vi "camera_acq_H_noshutter_sub.vi"(5 "Shutter time (ms)":dbl, 7 "Exposure time (ms)":dbl, 8 "error in (no error)":errorcluster, 9 "Binning":dbl=1.0 format="%#_13g", 10 "Camera in":u32, 11 "VISA in":refnum<visa-resource-name>) -> (0 "error out":errorcluster, 1 "Image":u16[][](graph), 2 "Camera out":u32, 3 "VISA out":refnum<visa-resource-name>)   [LabVIEW 2018]
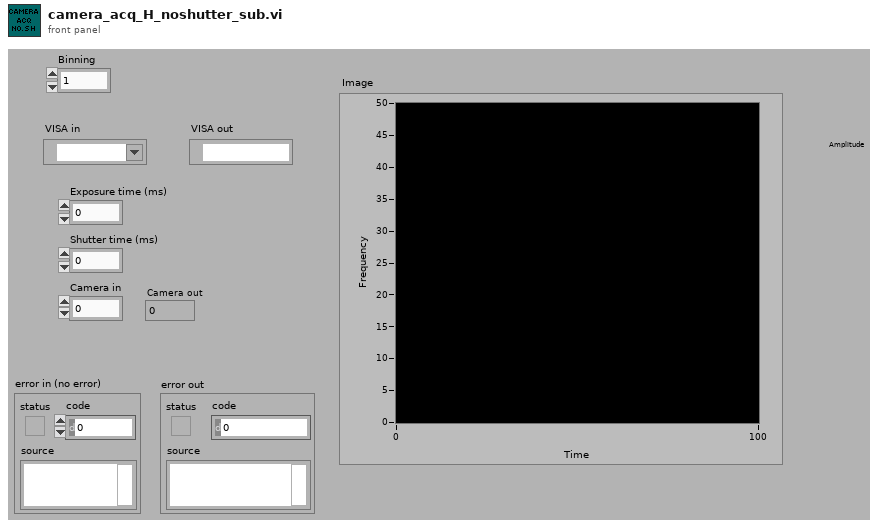
[diagram p1: front panel]
types:
  T1 = enum16{"Fast-mode", "Soft-mode", "Neutral Density"}
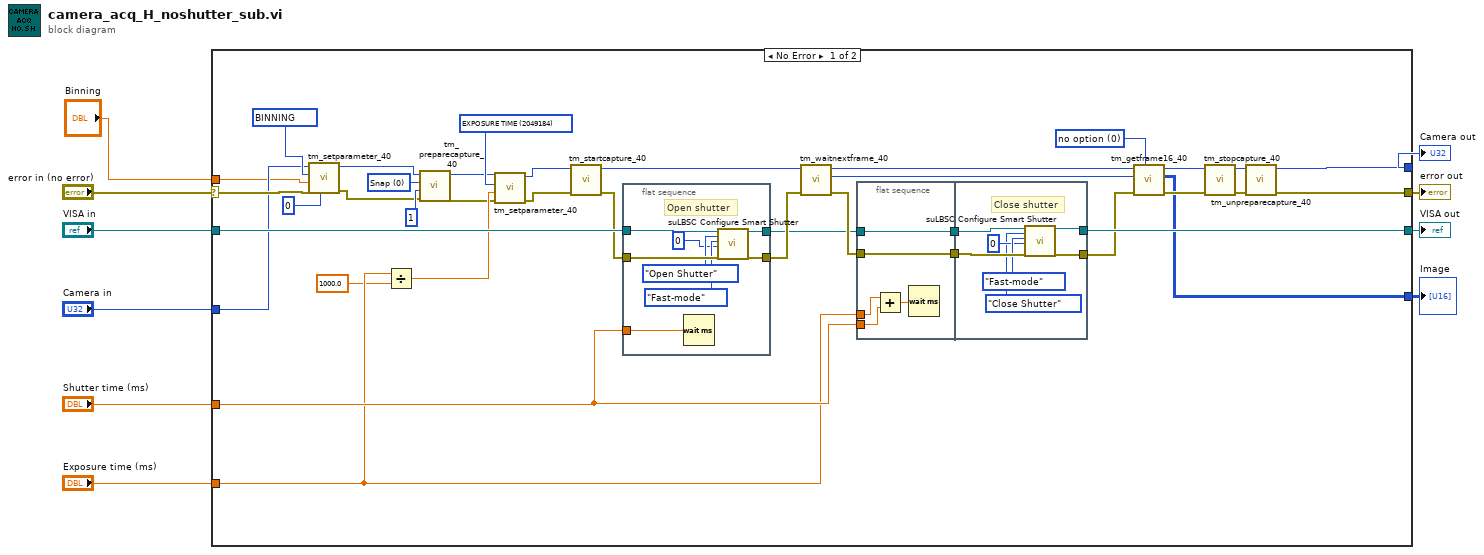
[diagram p0: block diagram]
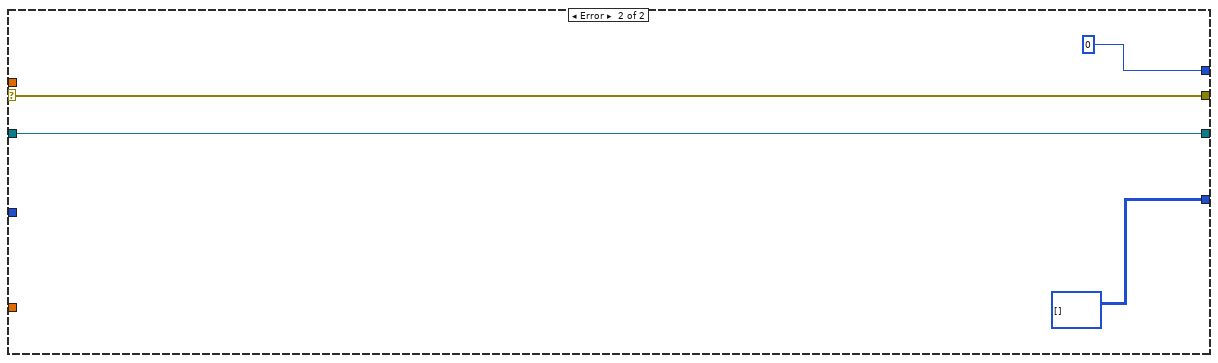
[diagram p2: hidden frame]
diagram:
  n1 = case shown="No Error" "error in (no error)" {
    selector: "error in (no error)" -> [w19 w71]
    tunnel: "Exposure time (ms)" -> [w31 _]
    tunnel: [w22 u32 0 ("Handle out")] -> w8
    tunnel: "VISA in" -> [w45 w72]
    tunnel: "Shutter time (ms)" -> [w44 _]
    tunnel: [w36 w71] -> w10
    tunnel: [w43 w72] -> w4
    tunnel: "Camera in" -> [w18 _]
    tunnel: [w32 u16[][] [] ("Data")] -> w2
    tunnel: "Binning" -> [w11 _]
    frame No Error {
      w16 = 0 items=["Snap", "Sequence"] ("Capture mode")
      w21 = u32 4215968 items=["SENSOR MODE"=4212128, "READOUT SPEED"=4211872, "READOUT DIRECTION"=4211904, "TRIGGER GLOBAL EXPOSURE"=2049680, "TRIGGER DELAY"=1066480, "INTERNAL TRIGGER HANDLING"=1066496, "SYNC READOUT SYSTEM BLANK"=1066528, "SENSOR TEMPERATURE"=2115232, "SENSOR COOLER STATUS"=2115280, "EXPOSURE TIME"=2049184, "DEFECT CORRECT MODE"=4670368, "BINNING"=4215968, "INTERNAL LINE SPEED"=4226000, "INTERNAL LINE INTERVAL"=4226016, "NUMBER OF OUTPUT TRIGGER CONNECTOR"=1852320, "OUTPUT TRIGGER SOURCE[0]"=1852576, "OUTPUT TRIGGER SOURCE[1]"=1852832, "OUTPUT TRIGGER SOURCE[2]"=1853088, "OUTPUT TRIGGER POLARITY[0]"=1852592, "OUTPUT TRIGGER POLARITY[1]"=1852848, "OUTPUT TRIGGER POLARITY[2]"=1853104, "OUTPUT TRIGGER ACTIVE[0]"=1852608, "OUTPUT TRIGGER ACTIVE[1]"=1852864, "OUTPUT TRIGGER ACTIVE[2]"=1853120, "OUTPUT TRIGGER DELAY[0]"=1852624, "OUTPUT TRIGGER DELAY[1]"=1852880, "OUTPUT TRIGGER DELAY[2]"=1853136, "OUTPUT TRIGGER PERIOD[0]"=1852640, "OUTPUT TRIGGER PERIOD[1]"=1852896, "OUTPUT TRIGGER PERIOD[2]"=1853152, "OUTPUT TRIGGER KIND[0]"=1852656, "OUTPUT TRIGGER KIND[1]"=1852912, "OUTPUT TRIGGER KIND[2]"=1853168, "OUTPUT TRIGGER BASE SENSOR[0]"=1852672, "OUTPUT TRIGGER BASE SENSOR[1]"=1852928, "OUTPUT TRIGGER BASE SENSOR[2]"=1853184, "OUTPUT TRIGGER PRE HSYNC COUNT"=1852704] ("Parameter")
      w26 = 0 items=["no option"=0, "high contrast"=16] ("Options")
      w42 = u32 2049184 items=["SENSOR MODE"=4212128, "READOUT SPEED"=4211872, "READOUT DIRECTION"=4211904, "TRIGGER GLOBAL EXPOSURE"=2049680, "TRIGGER DELAY"=1066480, "INTERNAL TRIGGER HANDLING"=1066496, "SYNC READOUT SYSTEM BLANK"=1066528, "SENSOR TEMPERATURE"=2115232, "SENSOR COOLER STATUS"=2115280, "EXPOSURE TIME"=2049184, "DEFECT CORRECT MODE"=4670368, "BINNING"=4215968, "INTERNAL LINE SPEED"=4226000, "INTERNAL LINE INTERVAL"=4226016, "NUMBER OF OUTPUT TRIGGER CONNECTOR"=1852320, "OUTPUT TRIGGER SOURCE[0]"=1852576, "OUTPUT TRIGGER SOURCE[1]"=1852832, "OUTPUT TRIGGER SOURCE[2]"=1853088, "OUTPUT TRIGGER POLARITY[0]"=1852592, "OUTPUT TRIGGER POLARITY[1]"=1852848, "OUTPUT TRIGGER POLARITY[2]"=1853104, "OUTPUT TRIGGER ACTIVE[0]"=1852608, "OUTPUT TRIGGER ACTIVE[1]"=1852864, "OUTPUT TRIGGER ACTIVE[2]"=1853120, "OUTPUT TRIGGER DELAY[0]"=1852624, "OUTPUT TRIGGER DELAY[1]"=1852880, "OUTPUT TRIGGER DELAY[2]"=1853136, "OUTPUT TRIGGER PERIOD[0]"=1852640, "OUTPUT TRIGGER PERIOD[1]"=1852896, "OUTPUT TRIGGER PERIOD[2]"=1853152, "OUTPUT TRIGGER KIND[0]"=1852656, "OUTPUT TRIGGER KIND[1]"=1852912, "OUTPUT TRIGGER KIND[2]"=1853168, "OUTPUT TRIGGER BASE SENSOR[0]"=1852672, "OUTPUT TRIGGER BASE SENSOR[1]"=1852928, "OUTPUT TRIGGER BASE SENSOR[2]"=1853184, "OUTPUT TRIGGER PRE HSYNC COUNT"=1852704] ("Parameter")
      n2 = call <userlib>:"tm_setparameter_40.vi"("Index"=0, "error in (no error)"=w19, "Value in"=w11, "Parameter"=w21, "Handle in"=w18) -> ("error out"=w12:errorcluster, "Handle out"=w15:u32)  [unwired: 5 in]
      n3 = Divide(x=w31, y=1000.0) -> (x/y=w23:dbl)
      n4 = call <userlib>:"tm_preparecapture_40.vi"("error in (no error)"=w12, "Frames"=1, "Capture mode"=w16, "Handle in"=w15) -> ("error out"=w13:errorcluster, "Handle out"=w14:u32)  [unwired: 4 in, 2 out]
      n5 = call <userlib>:"tm_setparameter_40.vi"("error in (no error)"=w13, "Value in"=w23, "Parameter"=w42, "Handle in"=w14) -> ("error out"=w24:errorcluster, "Handle out"=w25:u32)  [unwired: 6 in]
      n6 = call <userlib>:"tm_startcapture_40.vi"("error in (no error)"=w24, "Handle in"=w25) -> ("error out"=w27:errorcluster, "Handle out"=w41:u32)  [unwired: 8 in]
      n7 = flat-sequence {
        tunnel: w27 -> [w67]
        tunnel: w45 -> [w65]
        tunnel: w44 -> [w68]
        tunnel: [w66] -> w48
        tunnel: [w64] -> w28
        frame #0 {
          # "Open shutter"
          n8 = Wait (ms)(milliseconds to wait=w68) -> ()  [unwired: 1 out]
          n9 = call "suLBSC Configure Smart Shutter.vi"("VISA resource name"=w65, "SmartShutter State (0: Open Shutter)"=enum16{"Open Shutter", "Close Shutter"}."Open Shutter", "SmartShutter Mode (0: Fast-mode)"=T1."Fast-mode", "Neutral Density Microsteps (0)"=u8 0, "error in (no error)"=w67) -> ("VISA resource name  out"=w64:refnum<visa-resource-name>, "error out"=w66:errorcluster)  [unwired: 13 in]
        }
      }
      n10 = call <userlib>:"tm_waitnextframe_40.vi"("error in (no error)"=w48, "Handle in"=w41) -> ("error out"=w47:errorcluster, "Frame Index"=w33:i32, "Handle out"=w40:u32)  [unwired: 6 in, 1 out]
      n11 = flat-sequence {
        tunnel: w44 -> [w49]
        tunnel: w31 -> [w50]
        tunnel: w47 -> [w52]
        tunnel: [w52] -> w46
        tunnel: w28 -> [w51]
        tunnel: [w51] -> w29
        tunnel: w46 -> [w59]
        tunnel: [w55] -> w43
        tunnel: [w60] -> w39
        tunnel: w29 -> [w54]
        frame #0 {
          n12 = Add(x=w50, y=w49) -> (x+y=w53:dbl)
          n13 = Wait (ms)(milliseconds to wait=w53) -> ()  [unwired: 1 out]
        }
        frame #1 {
          # "Close shutter"
          n14 = call "suLBSC Configure Smart Shutter.vi"("VISA resource name"=w54, "SmartShutter State (0: Open Shutter)"=enum16{"Open Shutter", "Close Shutter"}."Close Shutter", "SmartShutter Mode (0: Fast-mode)"=T1."Fast-mode", "Neutral Density Microsteps (0)"=u8 0, "error in (no error)"=w59) -> ("VISA resource name  out"=w55:refnum<visa-resource-name>, "error out"=w60:errorcluster)  [unwired: 13 in]
        }
      }
      n15 = call <userlib>:"tm_getframe16_40.vi"("Options"=w26, "error in (no error)"=w39, "Frame Index"=w33, "Handle in"=w40) -> ("error out"=w38:errorcluster, "Data"=w32:u16[][], "Handle out"=w34:u32)  [unwired: 4 in, 1 out]
      n16 = call <userlib>:"tm_stopcapture_40.vi"("error in (no error)"=w38, "Handle in"=w34) -> ("error out"=w37:errorcluster, "Handle out"=w35:u32)  [unwired: 8 in]
      n17 = call <userlib>:"tm_unpreparecapture_40.vi"("error in (no error)"=w37, "Handle in"=w35) -> ("error out"=w36:errorcluster, "Handle out"=w22:u32)  [unwired: 8 in]
    }
    frame Error {
    }
  }
  "Camera out" <- w8
  "error out" <- w10
  "VISA out" <- w4
  "Image" <- w2
